vi "Logger.vi"(0 "Module Data In":T1, 5 "Log Process?":bool, 11 "error in (no error)":errorcluster) -> (4 "Module Data Out":T1, 15 "error out":errorcluster)   [LabVIEW 2020, in "Template.lvlib"]
doc: "Loggs states and processes as they are being handled by the module"
uses:
  Template.lvlib
  Controls/Module - Data.ctl
  Modules.ctl
  Controls/Module - States.ctl
  Controls/Timing - Data.ctl
  Controls/Process - Element.ctl
  Controls/Process.ctl
  Controls/Process - Status.ctl
  Error Handler - Logger Module/Error Handler - Logger.lvlib
panel:
  out "Log":string
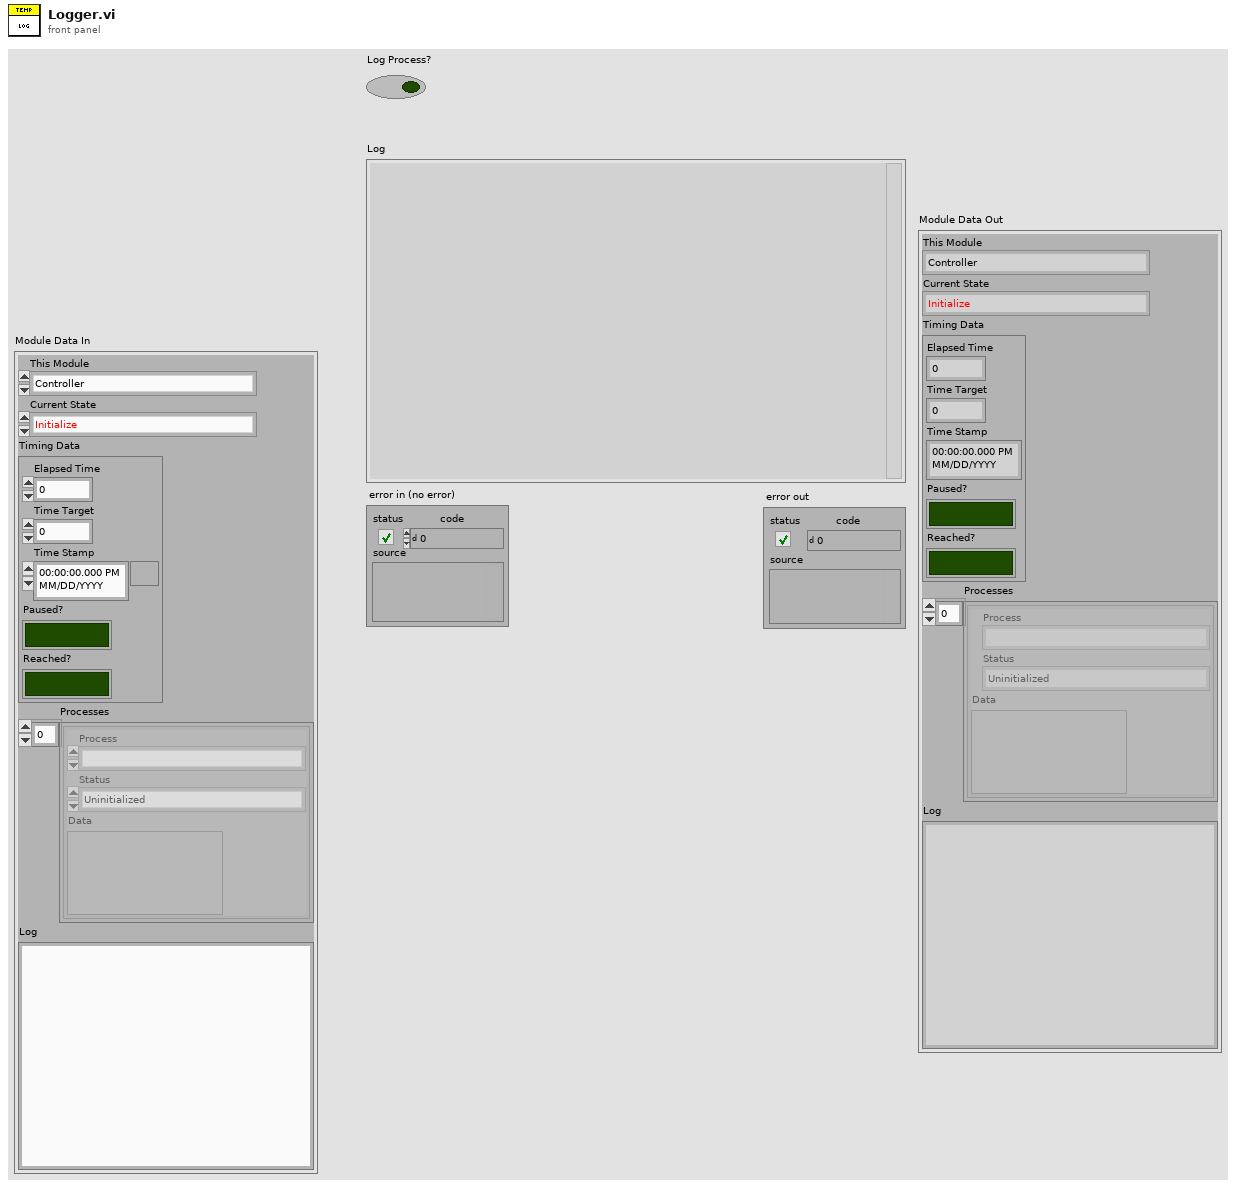
[diagram p1: front panel]
types:
  T1 = typedef "Template.lvlib/Module - Data.ctl" = cluster{"This Module":T2, "Current State":T3, "Timing Data":T4, "Processes":T5[], "Log":string}
  T2 = typedef "Error Handler - Logger.lvlib/Modules.ctl" = enum16{"Controller", "Error Handler - Logger"}
  T3 = typedef "Template.lvlib/Module - States.ctl" = enum16{"Initialize", "Event ", "Send data", "FP Element: Update", "FP Element: Disable/Enable", "Timer: Setup", "Terminate", "---------------Template---------------"}
  T4 = typedef "Template.lvlib/Timing - Data.ctl" = cluster{"Elapsed Time":dbl, "Time Target":dbl, "Time Stamp":timestamp, "Paused?":bool, "Reached?":bool}
  T5 = typedef "Template.lvlib/Process - Element.ctl" = cluster{"Process":T6, "Status":T7, "Data":variant}
  T6 = typedef "Template.lvlib/Process.ctl" = enum16{""}
  T7 = typedef "Template.lvlib/Process - Status.ctl" = enum16{"Uninitialized", "Busy"}
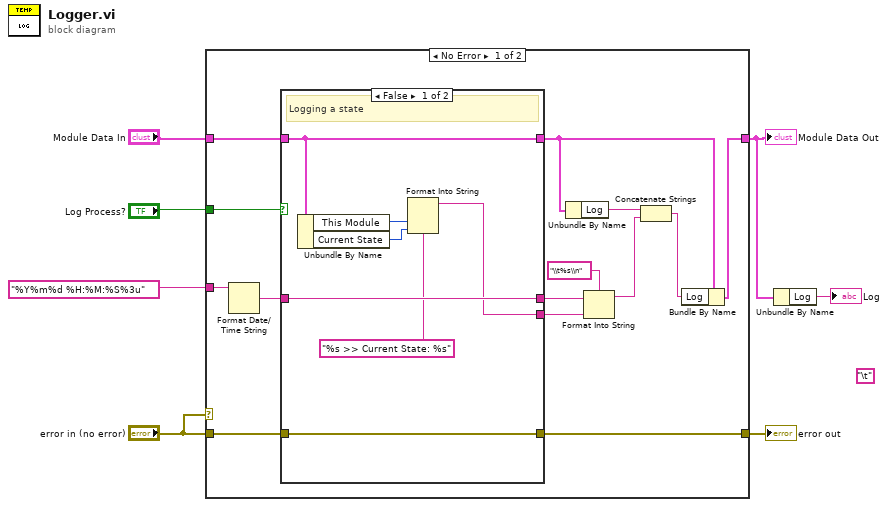
[diagram p0: block diagram]
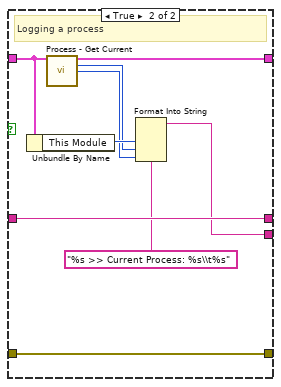
[diagram p2: hidden frame]
diagram:
  (unwired) "\t" ("format string")
  n1 = case shown="No Error" "error in (no error)" {
    tunnel: [w13 w39] -> w4
    tunnel: "Module Data In" -> [w21 w39]
    tunnel: [w19 w38] -> w6
    tunnel: "error in (no error)" -> [w20 w38]
    tunnel: "Log Process?" -> [w18 _]
    tunnel: "%Y%m%d %H:%M:%S%3u" ("time format string (%c)") -> [w12 _]
    frame No Error {
      n2 = Format Date/Time String(time format string (%c)=w12) -> (date/time string=w17:string)  [unwired: 2 in]
      n3 = case shown="False" w18 {
        tunnel: w21 -> [w27 w32]
        tunnel: [w27 w31] -> w11
        tunnel: w20 -> [w28 w37]
        tunnel: [w28 w37] -> w19
        tunnel: w17 -> [w26 w36]
        tunnel: [w26 w36] -> w16
        tunnel: [w25 w35] -> w15
        frame False {
          # "Logging a state"
          n4 = Unbundle By Name(w27) -> ("This Module"=w24:T2, "Current State"=w23:T3)
          n5 = Format Into String(format string="%s >> Current State: %s", w24, w23) -> (resulting string=w25:string)  [unwired: 2 in, 1 out]
        }
        frame True {
          # "Logging a process"
          n6 = Unbundle By Name(w32) -> ("This Module"=w34:T2)
          n7 = call "Process - Get Current.vi"("Module Data In"=w32) -> ("Module Data Out"=w31:T1, "Process"=w30:T6, "Status"=w29:T7)  [unwired: 9 in, 3 out]
          n8 = Format Into String(format string="%s >> Current Process: %s\\t%s", w34, w30, w29) -> (resulting string=w35:string)  [unwired: 2 in, 1 out]
        }
      }
      n9 = Unbundle By Name(w11) -> ("Log"=w10:string)
      n10 = Format Into String(format string="\\t%s\\n", initial string=w16, w15) -> (resulting string=w8:string)  [unwired: 1 in, 1 out]
      n11 = Concatenate Strings(w10, w8) -> (w9:string)
      n12 = Bundle By Name(cluster=w11, "Log"=w9) -> (w13:T1)
    }
    frame Error {
    }
  }
  "error out" <- w6
  "Module Data Out" <- w4
  n13 = Unbundle By Name(w4) -> ("Log"=→"Log":string)
